vi "DriveModuleReadEncoder.vi"(8 "error in":errorcluster, 11 "ModualNamePrefix":i32) -> (0 "error out":errorcluster, 2 "SWERVE_DRIVE_MODULE_POSITION":T1={"Distance"=0.0, "Angle"={"VALUE"=0.0, "COS"=1.0, "SIN"=0.0}, "P"=FALSE} {"Angle"."SIN" format="%13.4f"; "Angle"."COS" format="%13.4f"; "Angle"."VALUE" format="%13.4f"}, 3 "SWERVE_DRIVE_MODULE_STATE":T3={"Speed"=0.0, "Angle"={"VALUE"=0.0, "COS"=1.0, "SIN"=0.0}} {"Angle"."SIN" format="%13.4f"; "Angle"."COS" format="%13.4f"; "Angle"."VALUE" format="%13.4f"})   [LabVIEW 2023]
uses:
  <vilib>/Rock Robotics/WPI/ThirdParty/JAS_Junk/TrajLib/TypeDef/SWERVE_DRIVE_MODULE_STATE.ctl
  <vilib>/Rock Robotics/WPI/ThirdParty/JAS_Junk/TrajLib/TypeDef/ROTATION2D.ctl
  <vilib>/Rock Robotics/WPI/ThirdParty/JAS_Junk/TrajLib/TypeDef/SWERVE_DRIVE_MODULE_POSITION.ctl
  <vilib>/Rock Robotics/WPI/ThirdParty/JAS_Junk/TrajLib/Conv_Deg_Radians.vi
  <vilib>/Rock Robotics/WPI/ThirdParty/JAS_Junk/TrajLib/Rotation2d_CreateAngle.vi
  Drive/DriveGlobal.vi
  <vilib>/Rock Robotics/WPI/ThirdParty/Phoenix6/Phoenix6_Device_RefNumRegistryGet.vi
  <vilib>/Rock Robotics/WPI/MotorControl/WPI_MotorControlRefNum Registry Get.vi
  <vilib>/Rock Robotics/WPI/ThirdParty/Phoenix6/getters/GetCANcoder_AbsPosition.vi
  <vilib>/Rock Robotics/WPI/ThirdParty/Phoenix6/getters/GetCANcoder_Velocity.vi
  <vilib>/Rock Robotics/WPI/ThirdParty/Phoenix6/getters/GetCANcoder_Position.vi
  <vilib>/Rock Robotics/Network Tables/NT Write Number.vi
  <vilib>/Rock Robotics/WPI/ThirdParty/REV Robotics/REVLib/SubVI/Public/SPARK Get Encoder Status Position.vi
  <vilib>/Rock Robotics/WPI/ThirdParty/REV Robotics/REVLib/SubVI/Public/SPARK Get Encoder Status Velocity.vi
  <vilib>/Rock Robotics/WPI/ThirdParty/JAS_Junk/TrajLib/Trajectory_Library.lvlib
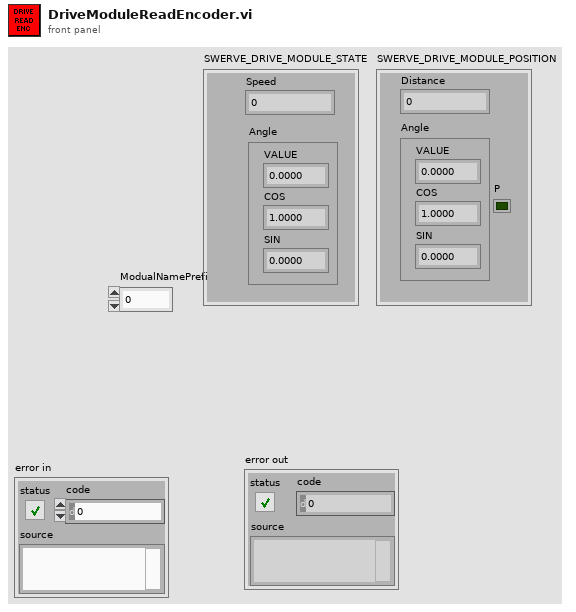
[diagram p1: front panel]
types:
  T1 = typedef "Trajectory_Library.lvlib/SWERVE_DRIVE_MODULE_POSITION.ctl" = cluster{"Distance":dbl, "Angle":T2, "P":bool}
  T2 = typedef "Trajectory_Library.lvlib/ROTATION2D.ctl" = cluster{"VALUE":dbl, "COS":dbl, "SIN":dbl}
  T3 = typedef "Trajectory_Library.lvlib/SWERVE_DRIVE_MODULE_STATE.ctl" = cluster{"Speed":dbl, "Angle":T2}
  T4 = typedef "WPI_MotorControlDeviceRef.ctl" = cluster{"DeviceStatus":errorcluster, "Type":T5, "PWM":cluster{"PWM Channel":T6, "DeadBand":T7}, "CAN":cluster{"Device Number":u8, "SetOutput VI Ref":variant, "GetOutput VI Ref":variant, "Enable VI Ref":variant, "Disable VI Ref":variant, "Data":variant}, "Invert":bool, "DIO PWM":cluster{"PWM \"Enable\" Channel":T6, "DIOChannel":T8, "PWM Rate":dbl}}
  T5 = typedef "WPI_MotorControlType.ctl" = enum16{"PWM", "CAN", "DIO PWM"}
  T6 = typedef "FPGA_DIOPWMChannel.ctl" = enum8{"PWM 0", "PWM 1", "PWM 2", "PWM 3", "PWM 4", "PWM 5", "PWM 6", "PWM 7", "PWM 8", "PWM 9", "PWM MXP 0", "PWM MXP 1", "PWM MXP 2", "PWM MXP 3", "PWM MXP 4", "PWM MXP 5", "PWM MXP 6", "PWM MXP 7", "PWM MXP 8", "PWM MXP 9", "Invalid"}
  T7 = typedef "WPI_PWMDeadband.ctl" = cluster{"Name":string, "maxPositivePwm":i32, "minPositivePwm":i32, "centerPwm":i32, "maxNegativePwm":i32, "minNegativePwm":i32, "angularRange":u16}
  T8 = typedef "FPGA_DIOChannel.ctl" = enum8{"DIO 0", "DIO 1", "DIO 2", "DIO 3", "DIO 4", "DIO 5", "DIO 6", "DIO 7", "DIO 8", "DIO 9", "DIO MXP 0", "DIO MXP 1", "DIO MXP 2", "DIO MXP 3", "DIO MXP 4", "DIO MXP 5", "DIO MXP 6", "DIO MXP 7", "DIO MXP 8", "DIO MXP 9", "DIO MXP 10", "DIO MXP 11", "DIO MXP 12", "DIO MXP 13", "DIO MXP 14", "DIO MXP 15", "SPI Port CS1", "SPI Port CS2", "SPI Port CS3", "SPI Port MISO", "SPI Port MOSI", "Invalid"}
  T9 = typedef "DeviceReference.ctl" = cluster{"CANbus Name":string, "Device Encoding":u32, "Device Name":string}
  T10 = cluster{"Value":dbl, "System Timestamp":dbl, "CANivore Timestamp":dbl, "ECU Timestamp":dbl}
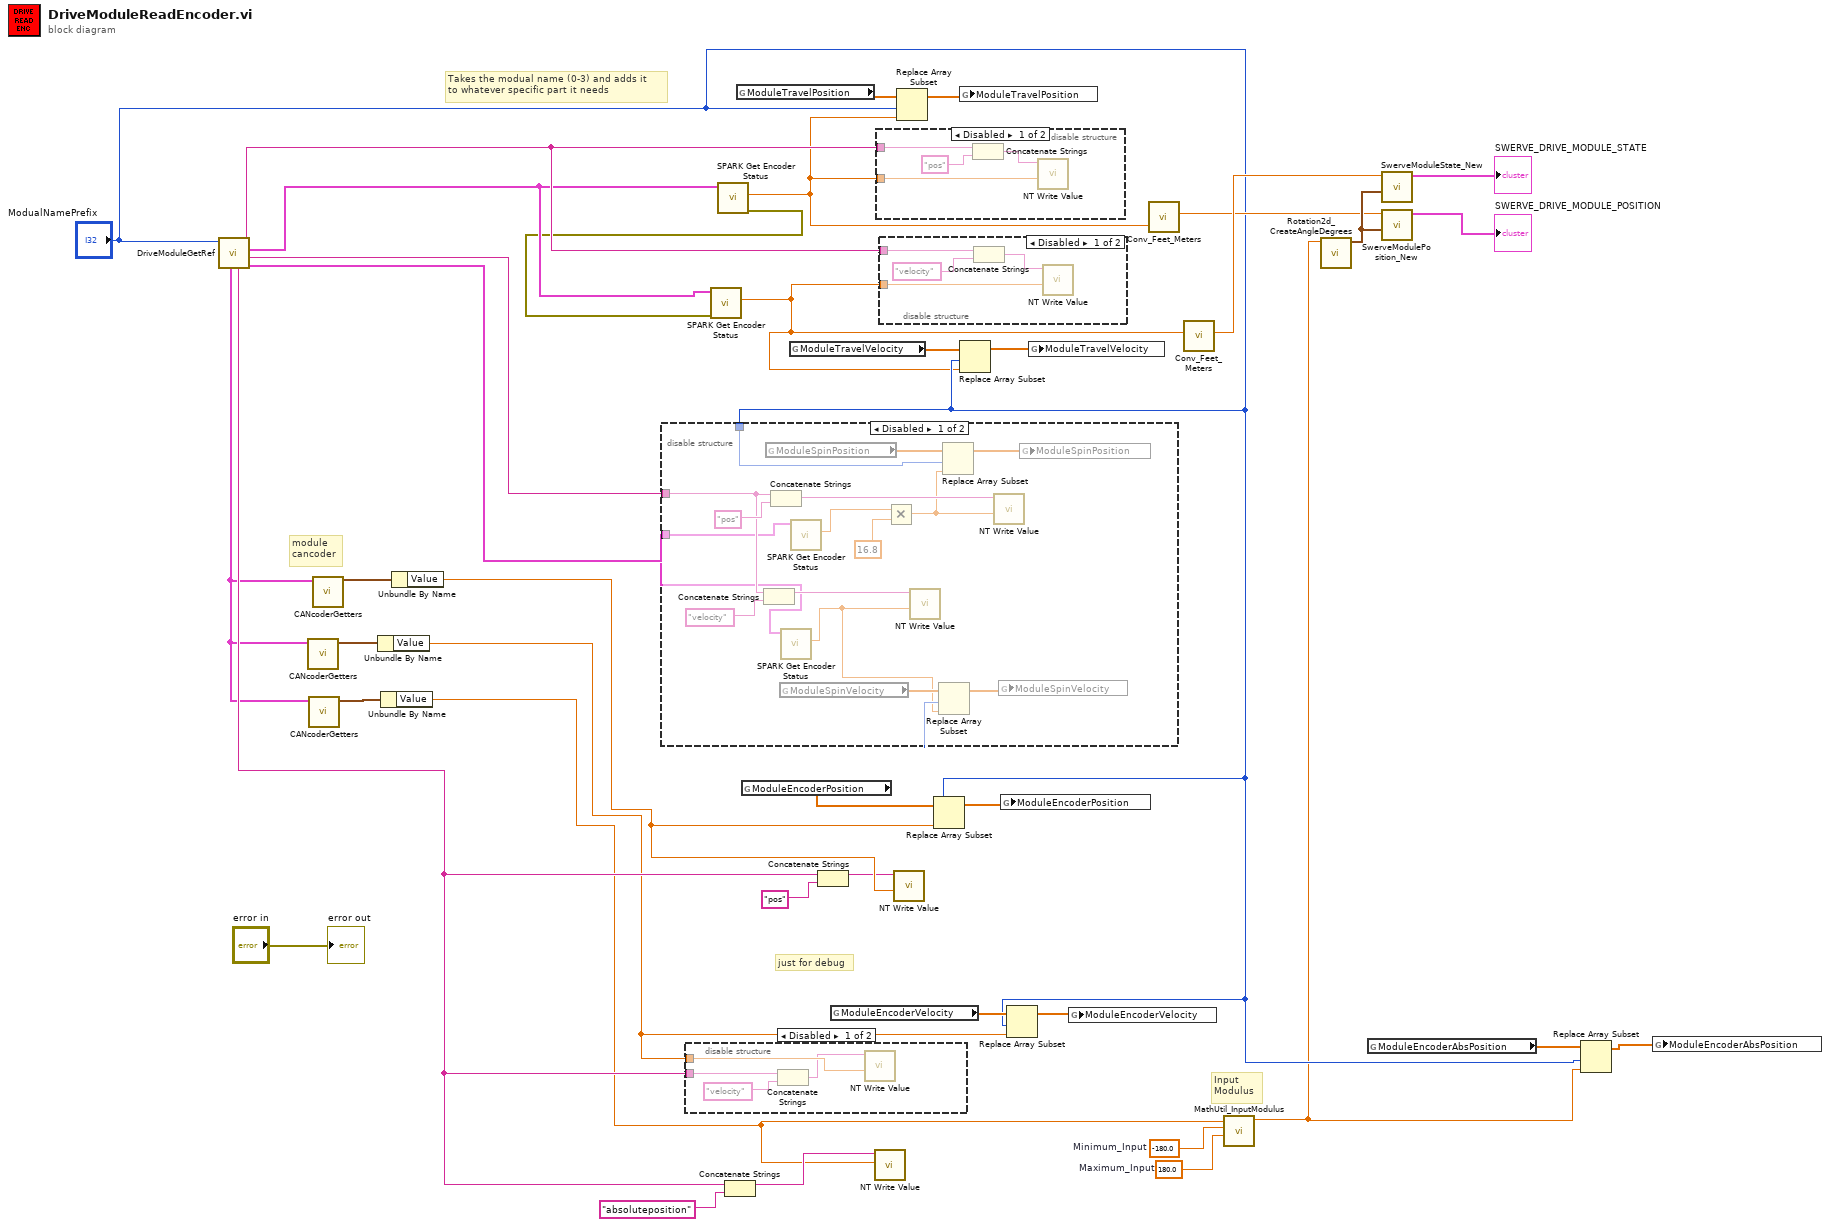
[diagram p0: block diagram]
diagram:
  w33 = -180.0  # Minimum_Input
  w32 = 180.0  # Maximum_Input
  # "module\ncancoder"
  # "Input\nModulus"
  # "just for debug"
  # "Takes the modual name (0-3) and adds it \nto whatever specific part it needs"
  n1 = call "DriveModuleGetRef.vi"("ModualNamePrefix"="ModualNamePrefix") -> ("SpinMot"=w25:T4, "SpinStr"=w27:string, "TravMot"=w12:T4, "TravStr"=w26:string, "EncStr"=w24:string, "SpinEncRef"=w9:T9)  [unwired: 5 in]
  n2 = call-poly <vilib>:"CANcoderGetters.vi"("DeviceReference"=w9) -> ("Output"=w6:T10)  [unwired: 9 in, 1 out]
  n3 = call-poly <vilib>:"CANcoderGetters.vi"("DeviceReference"=w9) -> ("Output"=w7:T10)  [unwired: 9 in, 1 out]
  n4 = call-poly <vilib>:"CANcoderGetters.vi"("DeviceReference"=w9) -> ("Output"=w8:T10)  [unwired: 9 in, 1 out]
  n5 = Unbundle By Name(w6) -> ("Value"=w4:dbl)
  n6 = Unbundle By Name(w7) -> ("Value"=w3:dbl)
  n7 = Unbundle By Name(w8) -> ("Value"=w5:dbl)
  n8 = disable-structure shown="Disabled" {
    disable-tunnel: w27 -> [w49 _]
    disable-tunnel: w25 -> [w41 _]
    disable-tunnel: "ModualNamePrefix" -> [w43 _]
    frame Disabled {
      n9 = Concatenate Strings(w49, "velocity" ("refnum name")) -> (w51:string)
      n10 = global read "DriveGlobal.vi" "ModuleSpinPosition"() -> (w48:dbl[])
      n11 = Concatenate Strings(w49, "pos" ("refnum name")) -> (w53:string)
      n12 = global read "DriveGlobal.vi" "ModuleSpinVelocity"() -> (w45:dbl[])
      n13 = call-poly <vilib>:"SPARK Get Encoder Status.vi"("MotorControlDevRef in"=w41) -> ("Sensor Velocity"=w40:dbl)  [unwired: 7 in, 3 out]
      n14 = call-poly <vilib>:"SPARK Get Encoder Status.vi"("MotorControlDevRef in"=w41) -> ("Sensor Position"=w42:dbl)  [unwired: 7 in, 3 out]
      n15 = Multiply(x=w42, y=16.8) -> (x*y=w46:dbl)
      n16 = call-poly <vilib>:"NT Write Value.vi"("value"=w40, "name"=w51) -> ()  [unwired: 9 in, 1 out]
      n17 = Replace Array Subset(array=w45, new element=w40, index=w43) -> (w44:dbl[])
      n18 = Replace Array Subset(array=w48, new element=w46, index=w43) -> (w47:dbl[])
      n19 = call-poly <vilib>:"NT Write Value.vi"("value"=w46, "name"=w53) -> ()  [unwired: 9 in, 1 out]
      n20 = global write "DriveGlobal.vi" "ModuleSpinVelocity"(w44) -> ()
      n21 = global write "DriveGlobal.vi" "ModuleSpinPosition"(w47) -> ()
    }
    frame Enabled {
    }
  }
  n22 = disable-structure shown="Disabled" {
    disable-tunnel: w24 -> [w58 _]
    disable-tunnel: w4 -> [w57 _]
    frame Disabled {
      n23 = Concatenate Strings(w58, "velocity" ("refnum name")) -> (w55:string)
      n24 = call-poly <vilib>:"NT Write Value.vi"("value"=w57, "name"=w55) -> ()  [unwired: 9 in, 1 out]
    }
    frame Enabled {
    }
  }
  n25 = call-poly <vilib>:"SPARK Get Encoder Status.vi"("MotorControlDevRef in"=w12) -> ("error out"=w10:errorcluster, "Sensor Position"=w13:dbl)  [unwired: 7 in, 2 out]
  n26 = call-poly <vilib>:"SPARK Get Encoder Status.vi"("error in (no error)"=w10, "MotorControlDevRef in"=w12) -> ("Sensor Velocity"=w11:dbl)  [unwired: 6 in, 3 out]
  n27 = Concatenate Strings(w24, "absoluteposition" ("refnum name")) -> (w37:string)
  n28 = global read "DriveGlobal.vi" "ModuleTravelPosition"() -> (w29:dbl[])
  n29 = global read "DriveGlobal.vi" "ModuleEncoderPosition"() -> (w21:dbl[])
  n30 = global read "DriveGlobal.vi" "ModuleTravelVelocity"() -> (w23:dbl[])
  n31 = Concatenate Strings(w24, "pos" ("refnum name")) -> (w1:string)
  n32 = global read "DriveGlobal.vi" "ModuleEncoderVelocity"() -> (w19:dbl[])
  n33 = call-poly <vilib>:"NT Write Value.vi"("value"=w3, "name"=w37) -> ()  [unwired: 9 in, 1 out]
  n34 = disable-structure shown="Disabled" {
    disable-tunnel: w26 -> [w60 _]
    disable-tunnel: w13 -> [w59 _]
    frame Disabled {
      n35 = Concatenate Strings(w60, "pos" ("refnum name")) -> (w61:string)
      n36 = call-poly <vilib>:"NT Write Value.vi"("value"=w59, "name"=w61) -> ()  [unwired: 9 in, 1 out]
    }
    frame Enabled {
    }
  }
  n37 = disable-structure shown="Disabled" {
    disable-tunnel: w26 -> [w64 _]
    disable-tunnel: w11 -> [w63 _]
    frame Disabled {
      n38 = Concatenate Strings(w64, "velocity" ("refnum name")) -> (w65:string)
      n39 = call-poly <vilib>:"NT Write Value.vi"("value"=w63, "name"=w65) -> ()  [unwired: 9 in, 1 out]
    }
    frame Enabled {
    }
  }
  n40 = call-poly <vilib>:"NT Write Value.vi"("value"=w5, "name"=w1) -> ()  [unwired: 9 in, 1 out]
  n41 = Replace Array Subset(array=w29, new element=w13, index="ModualNamePrefix") -> (w28:dbl[])
  n42 = Replace Array Subset(array=w21, new element=w5, index="ModualNamePrefix") -> (w20:dbl[])
  n43 = global write "DriveGlobal.vi" "ModuleTravelPosition"(w28) -> ()
  n44 = Replace Array Subset(array=w23, new element=w11, index="ModualNamePrefix") -> (w22:dbl[])
  n45 = global write "DriveGlobal.vi" "ModuleEncoderPosition"(w20) -> ()
  n46 = Replace Array Subset(array=w19, new element=w4, index="ModualNamePrefix") -> (w18:dbl[])
  n47 = global write "DriveGlobal.vi" "ModuleTravelVelocity"(w22) -> ()
  n48 = global write "DriveGlobal.vi" "ModuleEncoderVelocity"(w18) -> ()
  n49 = call <vilib>:"Conv_Feet_Meters.vi"("Feet"=w13) -> ("Meters"=w30:dbl)  [unwired: 10 in]
  n50 = call <vilib>:"Conv_Feet_Meters.vi"("Feet"=w11) -> ("Meters"=w31:dbl)  [unwired: 10 in]
  n51 = call <vilib>:"MathUtil_InputModulus.vi"("Maximum_Input"=w32, "Minimum_Input"=w33, "Input"=w3) -> ("modulus"=w14:dbl)  [unwired: 8 in]
  n52 = call <vilib>:"Rotation2d_CreateAngleDegrees.vi"("Angle_Degrees"=w14) -> ("ROTATION"=w36:T2)  [unwired: 10 in]
  n53 = global read "DriveGlobal.vi" "ModuleEncoderAbsPosition"() -> (w17:dbl[])
  n54 = call <vilib>:"SwerveModuleState_New.vi"("ROTATION"=w36, "Speed"=w31) -> ("SWERVE_DRIVE_MODULE_STATE"=→"SWERVE_DRIVE_MODULE_STATE":T3)  [unwired: 9 in]
  n55 = call <vilib>:"SwerveModulePosition_New.vi"("ROTATION"=w36, "Distance"=w30) -> ("SWERVE_DRIVE_MODULE_POSITION"=→"SWERVE_DRIVE_MODULE_POSITION":T1)  [unwired: 9 in]
  n56 = Replace Array Subset(array=w17, new element=w14, index="ModualNamePrefix") -> (w16:dbl[])
  n57 = global write "DriveGlobal.vi" "ModuleEncoderAbsPosition"(w16) -> ()
  "error out" <- "error in"
